vi "428_COMM (SubVI).vi"(0 "VISA resource name":refnum<visa-resource-name>="COM4", 5 "Input\nbuffer size":u32=4096, 7 "End read on termination character?":bool=TRUE, 8 "End write with termination character?":bool=TRUE, 9 "termination char\n(0xA = '\\n' = LF)":u8=10 format="%.0x", 10 "flow control":u16(ring) items=["None", "On"], 11 "timeout (ms)":u32=5000, 12 "baud rate":u32=921600, 13 "data bits":u16=8 min=5 max=8 step=1, 14 "parity":u16(ring) items=["None", "Odd", "Even", "Mark", "Space"], 15 "stop bits":u16(ring)=10 items=["1.0"=10, "1.5"=15, "2.0"=20]) -> (4 "VISA resource name out":refnum<visa-resource-name>, 6 "error out":errorcluster)   [LabVIEW 2016]
uses:
  <vilib>/Instr/_visa.llb/VISA Configure Serial Port (Instr).vi
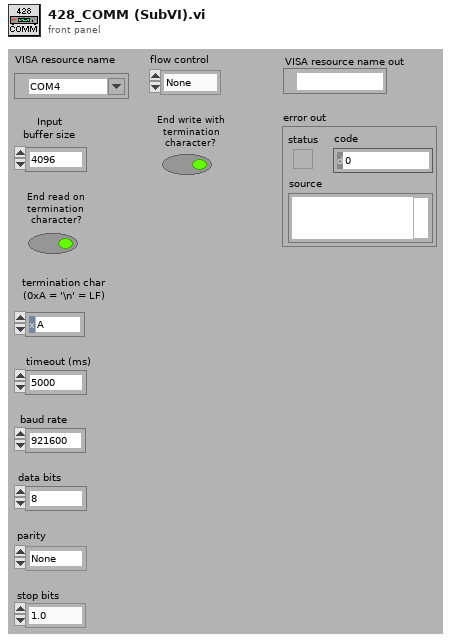
[diagram p1: front panel]
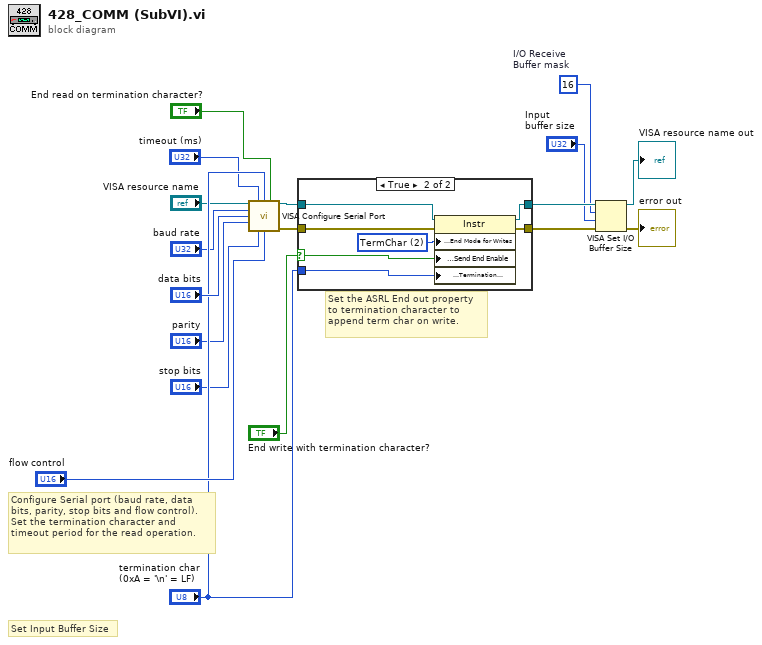
[diagram p0: block diagram]
diagram:
  w7 = u16 16  # I/O Receive Buffer mask
  # "Configure Serial port (baud rate, data\nbits, parity, stop bits and flow control).\nSet the termination character and\ntimeout period for the read operation."
  # "Set Input Buffer Size"
  # "Set the ASRL End out property\nto termination character to\nappend term char on write."
  n1 = call-poly "VISA Configure Serial Port"("VISA resource name"="VISA resource name", "timeout (10sec)"="timeout (ms)", "termination char\n(0xA = '\\n' = LF)"="termination char\n(0xA = '\\n' = LF)", "Enable Termination\nChar (T)"="End read on termination character?", "baud rate (9600)"="baud rate", "data bits (8)"="data bits", "parity (0:none)"="parity", "stop bits (10: 1 bit)"="stop bits", "flow control (0:none)"="flow control") -> ("VISA resource name out"=w15:refnum<visa-resource-name>, "error out"=w12:errorcluster)  [unwired: 5 in]
  n2 = case shown="True" "End write with termination character?" {
    selector: "End write with termination character?" -> [_ w21]
    tunnel: w15 -> [w19 w27]
    tunnel: w12 -> [w20 w26]
    tunnel: [w19 w25] -> w14
    tunnel: [w20 w24] -> w13
    tunnel: "termination char\n(0xA = '\\n' = LF)" -> [_ w22]
    frame False {
    }
    frame True {
      w23 = u16 2 items=["None", "LastBit", "TermChar", "Break"] ("Serial Settings:Serial End Mode for Writes")
      n3 = property class="Instr"(reference=w27, error in=w26, "Serial Settings:End Mode for Writes"=w23, "Message Based Settings:Send End Enable"=w21, "Message Based Settings:Termination Character"=w22) -> (reference out=w25:refnum<visa-resource-name>, error out=w24:errorcluster)
    }
  }
  n4 = VISA Set I/O Buffer Size(VISA resource name=w14, mask (16)=w7, size (4096)="Input\nbuffer size", error in (no error)=w13) -> (VISA resource name out=→"VISA resource name out":refnum<visa-resource-name>, error out=→"error out":errorcluster)
